vi "Refresh Tag Exchange Tab.vi"(6 "Tag Exchange Tab References":T1, 7 "Filter":string, 8 "error in (no error)":errorcluster, 10 "engine":refnum<data-value>, 11 "E2E editor node in":refnum<data-value>) -> (0 "error out":errorcluster, 2 "engine out":refnum<data-value>, 3 "E2E editor node out":refnum<data-value>)   [LabVIEW 2015, in "E2E Tag Exchange editor node.lvclass"]
uses:
  E2E Tag Exchange editor node.lvclass
  <vilib>/NI/DCAF/Tag Editor Core/Configuration Editor/Classes/Engine Parent/Engine Parent Editor Node.lvclass
  Tag Exchange Tab References.ctl
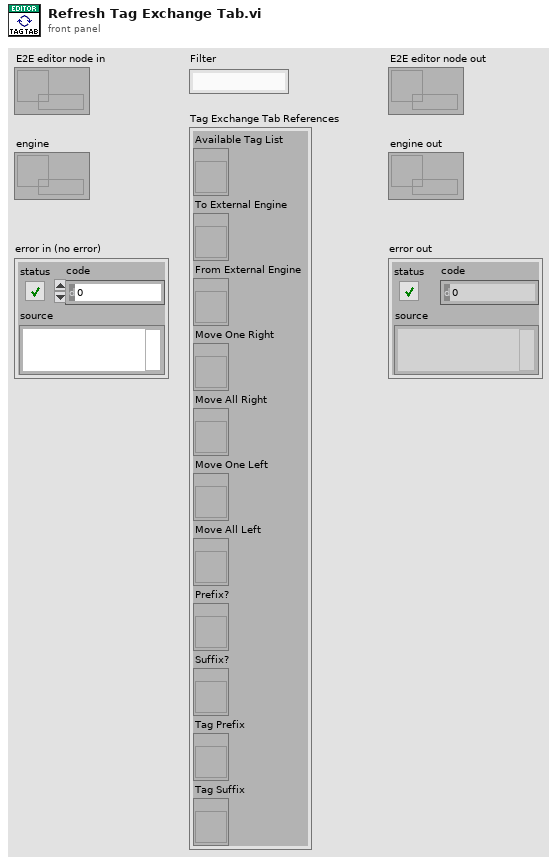
[diagram p1: front panel]
types:
  T1 = typedef "E2E Tag Exchange editor node.lvclass/Tag Exchange Tab References.ctl" = cluster{"Available Tag List":refnum<vi>, "To External Engine":refnum<vi>, "From External Engine":refnum<vi>, "Move One Right":refnum<vi>, "Move All Right":refnum<vi>, "Move One Left":refnum<vi>, "Move All Left":refnum<vi>, "Prefix?":refnum<vi>, "Suffix?":refnum<vi>, "Tag Prefix":refnum<vi>, "Tag Suffix":refnum<vi>}
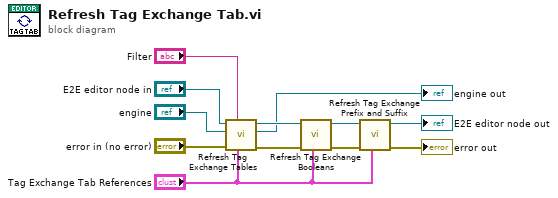
[diagram p0: block diagram]
diagram:
  n1 = call "Refresh Tag Exchange Tables.vi"("Tag Exchange Tab References"="Tag Exchange Tab References", "Filter"="Filter", "error in (no error)"="error in (no error)", "engine"="engine", "E2E editor node in"="E2E editor node in") -> ("error out"=w2:errorcluster, "engine out"=→"engine out":refnum<data-value>, "E2E editor node out"=w5:refnum<data-value>)  [unwired: 4 in]
  n2 = call "Refresh Tag Exchange Booleans.vi"("Tag Exchange Tab References"="Tag Exchange Tab References", "error in (no error)"=w2, "E2E editor node in"=w5) -> ("error out"=w7:errorcluster, "E2E editor node out"=w4:refnum<data-value>)  [unwired: 7 in]
  n3 = call "Refresh Tag Exchange Prefix and Suffix.vi"("Tag Exchange Tab References"="Tag Exchange Tab References", "error in (no error)"=w7, "E2E editor node in"=w4) -> ("error out"=→"error out":errorcluster, "E2E editor node out"=→"E2E editor node out":refnum<data-value>)  [unwired: 7 in]
